vi "SP Determine Ports to be De-embedded.vi"(9 "Measured Parameters":T1[](array[typedef]) {"Stimulus Port" min=1 step=1; "Response Port" min=1 step=1}, 10 "Adapters":T2[](array[typedef])) -> (1 "Ports to De-Embed":i8[](array[numeric]), 2 "Parameters to De-Embed":T1[](array[typedef]) {"Stimulus Port" min=1 step=1; "Response Port" min=1 step=1})   [LabVIEW 2011]
uses:
  TypeDefs/SP Adapter.ctl
  TypeDefs/SP Data.ctl
  TypeDefs/SP Parameter.ctl
  Summitek EXT/OpenG EXT/array/array.llb/Remove Duplicates from 1D Array (I8)__ogtk.vi
  Summitek EXT/OpenG EXT/array/array.llb/Filter 1D Array with Scalar (I8)__ogtk.vi
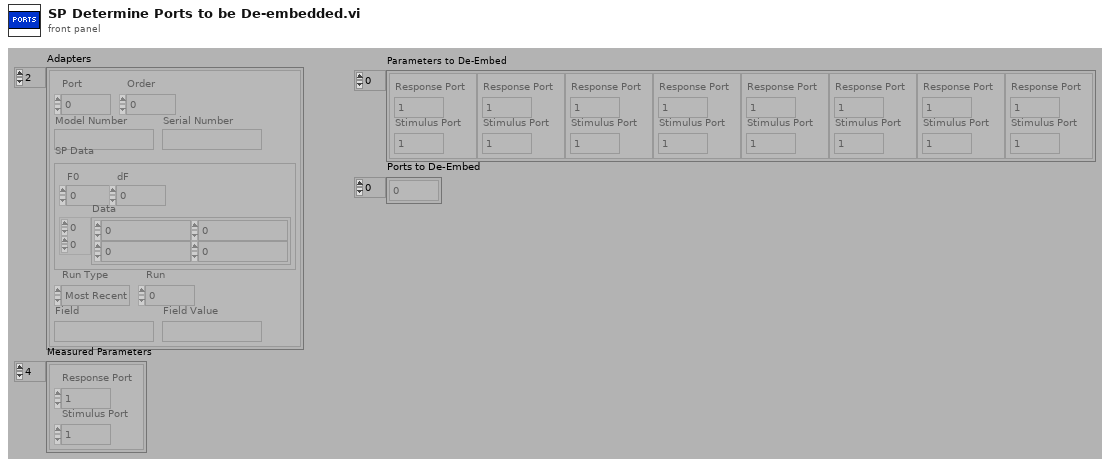
[diagram p1: front panel]
types:
  T1 = typedef "SP Parameter.ctl" = cluster{"Stimulus Port":i8, "Response Port":i8}
  T2 = typedef "SP Adapter.ctl" = cluster{"Port":i8, "Order":i8, "Model Number":string, "Serial Number":string, "SP Data":T3, "Run Type":enum16{"Most Recent", "Run #", "Match Field"}, "Run":i32, "Field":string, "Field Value":string}
  T3 = typedef "SP Data.ctl" = cluster{"F0":dbl, "dF":dbl, "Data":cdb[][]}
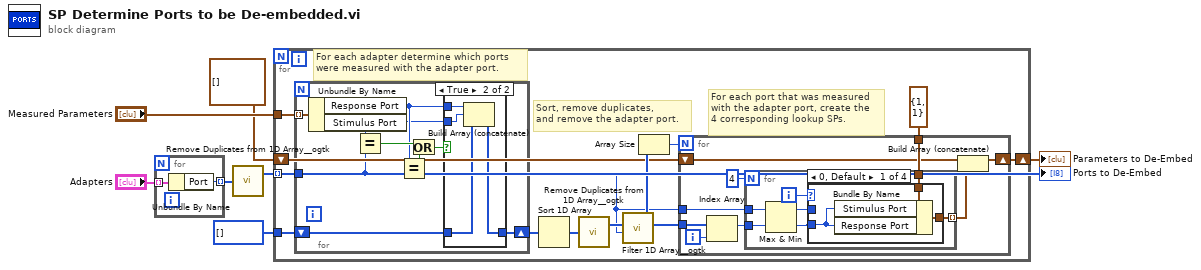
[diagram p0: block diagram]
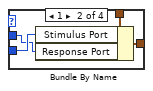
[diagram p2: hidden frame]
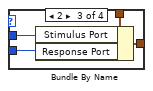
[diagram p3: hidden frame]
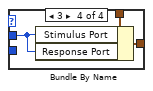
[diagram p4: hidden frame]
diagram:
  n1 = for {
    tunnel: "Adapters" -> [w9] mode=indexing
    tunnel: [w8] -> w6 mode=indexing
    n2 = Unbundle By Name(w9) -> ("Port"=w8:i8)
  }
  n3 = call-poly "Remove Duplicates from 1D Array__ogtk.vi"("Input Array"=w6) -> ("Output Array"=w4:i8[])  [unwired: 1 out]
  "Ports to De-Embed" <- w4
  n4 = for {
    tunnel: w4 -> [w10] mode=indexing
    tunnel: "Measured Parameters" -> [w20]
    shift-right: [w13] -> w3
    shift-left: T1[] [] ("Measured Parameters") -> [w11]
    tunnel: i8[] [] ("Output Array") -> [w12]
    # "For each adapter determine which ports\nwere measured with the adapter port."
    # "For each port that was measured\nwith the adapter port, create the\n4 corresponding lookup SPs."
    # "Sort, remove duplicates,\nand remove the adapter port."
    n5 = for {
      tunnel: w20 -> [w59] mode=indexing
      tunnel: w10 -> [w58]
      shift-right: [w51] -> w14
      shift-left: w12 -> [w54]
      n6 = Unbundle By Name(w59) -> ("Response Port"=w53:i8, "Stimulus Port"=w52:i8)
      n7 = Equal?(x=w52, y=w58) -> (x = y?=w56:bool)
      n8 = Equal?(x=w53, y=w58) -> (x = y?=w57:bool)
      n9 = Or(x=w56, y=w57) -> (x .or. y?=w55:bool)
      n10 = case shown="True" w55 {
        tunnel: w54 -> [w60 w62]
        tunnel: w53 -> [_ w64]
        tunnel: w52 -> [_ w63]
        tunnel: [w60 w61] -> w51
        frame False {
        }
        frame True {
          n11 = Build Array (concatenate)(w64, w63, w62) -> (w61:i8[])
        }
      }
    }
    n12 = Sort 1D Array(array=w14) -> (sorted array=w17:i8[])
    n13 = call-poly "Remove Duplicates from 1D Array__ogtk.vi"("Input Array"=w17) -> ("Output Array"=w18:i8[])  [unwired: 1 out]
    n14 = call-poly "Filter 1D Array__ogtk.vi"("items to filter"=w10, "array"=w18) -> ("filtered array"=w19:i8[])  [unwired: 5 out]
    n15 = Array Size(array=w19) -> (size(s)=w15:i32)
    n16 = for {
      N: w15 -> [_]
      tunnel: T1 {"Stimulus Port"=1, "Response Port"=1} ("Parameter") -> [w29]
      tunnel: w10 -> [w28]
      tunnel: w19 -> [w26]
      shift-right: [w22] -> w13
      shift-left: w11 -> [w24]
      i -> [w21]
      n17 = Index Array(array=w26, index=w21) -> (element=w25:i8)
      n18 = for {
        N: 4 -> [_]
        tunnel: w29 -> [w36]
        tunnel: w28 -> [w33]
        tunnel: w25 -> [w32]
        tunnel: [w34] -> w23 mode=indexing
        i -> [w35]
        n19 = Max & Min(x=w33, y=w32) -> (max(x,y)=w30:i8, min(x,y)=w31:i8)
        n20 = case shown="0, Default" w35 {
          tunnel: w36 -> [w39 w43 w47 w50]
          tunnel: w30 -> [_ w41 w46 w48]
          tunnel: w31 -> [w37 w42 w45 _]
          tunnel: [w38 w40 w44 w49] -> w34
          frame 0, Default {
            n21 = Bundle By Name(cluster=w39, "Stimulus Port"=w37, "Response Port"=w37) -> (w38:T1)
          }
          frame 1 {
            n22 = Bundle By Name(cluster=w43, "Stimulus Port"=w42, "Response Port"=w41) -> (w40:T1)
          }
          frame 2 {
            n23 = Bundle By Name(cluster=w47, "Stimulus Port"=w46, "Response Port"=w45) -> (w44:T1)
          }
          frame 3 {
            n24 = Bundle By Name(cluster=w50, "Stimulus Port"=w48, "Response Port"=w48) -> (w49:T1)
          }
        }
      }
      n25 = Build Array (concatenate)(w24, w23) -> (w22:T1[])
    }
  }
  "Parameters to De-Embed" <- w3
